vi "Heat2D_Interpolate 1D.vi"(10 "method":i32(ring)=1 items=["nearest", "linear", "spline", "cubic Hermite", "Lagrange"], 11 "X":dbl[](array[numeric])) -> (3 "Interp(X)":dbl[](array[numeric]))   [LabVIEW 2020, in "NI_PDE.lvlib"]
uses:
  <vilib>/gmath/NI_PDE.lvlib
  <vilib>/Analysis/1siggen.llb/Ramp Pattern by Samples.vi
  <vilib>/gmath/NI_Gmath.lvlib
  <vilib>/Analysis/NI_AALBase.lvlib
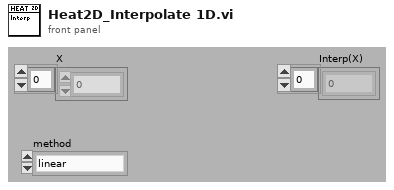
[diagram p1: front panel]
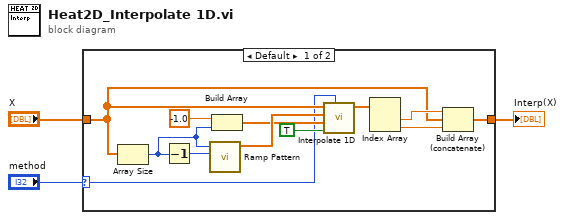
[diagram p0: block diagram]
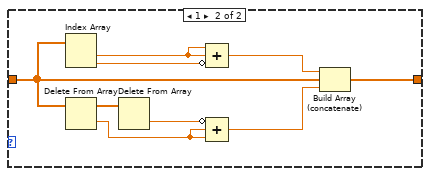
[diagram p2: hidden frame]
diagram:
  n1 = case shown="Default" "method" {
    selector: "method" -> [w4 _]
    tunnel: "X" -> [w6 w17]
    tunnel: [w5 w16] -> w2
    frame Default {
      n2 = Array Size(array=w6) -> (size(s)=w14:i32)
      n3 = Decrement(x=w14) -> (x-1=w10:i32)
      n4 = call-poly <vilib>:"Ramp Pattern.vi"("end"=w10, "samples"=w14) -> ("Ramp Pattern"=w9:dbl[])  [unwired: 8 in, 1 out]
      n5 = Build Array(-1.0 ("element"), w14) -> (w7:dbl[])
      n6 = call <vilib>:"Interpolate 1D.vi"("method"=w4, "X is monotonic"=TRUE, "xi"=w7, "X"=w9, "Y"=w6) -> ("yi"=w11:dbl[])  [unwired: 1 in, 5 out]
      n7 = Index Array(array=w11) -> (element #1=w12:dbl, element #2=w13:dbl)  [unwired: 2 in]
      n8 = Build Array (concatenate)(w12, w6, w13) -> (w5:dbl[])
    }
    frame 1 {
      n9 = Index Array(array=w17) -> (element #1=w19:dbl, element #2=w24:dbl)  [unwired: 2 in]
      n10 = Delete From Array(array=w17) -> (deleted portion=w21:dbl, array with subset deleted=w22:dbl[])  [unwired: 2 in]
      n11 = Delete From Array(array=w22) -> (deleted portion=w18:dbl)  [unwired: 2 in, 1 out]
      n12 = Compound Arithmetic op=ADD(w19, w19, invert w24) -> (w23:dbl)
      n13 = Compound Arithmetic op=ADD(invert w18, w21, w21) -> (w20:dbl)
      n14 = Build Array (concatenate)(w23, w17, w20) -> (w16:dbl[])
    }
  }
  "Interp(X)" <- w2
